vi "PH_AxisGUI_BaseClass.set Activity to GUI.vi"(4 "error in":errorcluster, 5 "no link":bool, 6 "Activity":T1, 7 "GUI Ref Activity":refnum<vi>) -> (0 "error out":errorcluster)   [LabVIEW 2014, in "PH_AxisGUI_BaseClass.lvlib"]
doc: "This VI sets the current activity to the GUI."
uses:
  PH_AxisGUI_BaseClass.lvlib
  PH_Stepmotor_BaseClass/PH_Stepmotor_BaseClass.Axis Activity.ctl
  PH_Stepmotor_BaseClass/PH_Stepmotor_BaseClass.lvlib
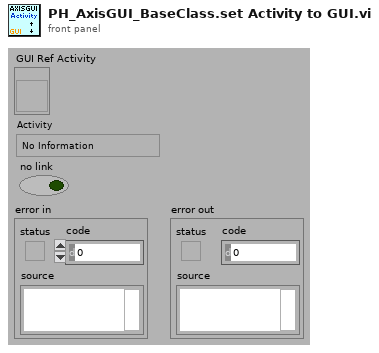
[diagram p1: front panel]
types:
  T1 = typedef "PH_Stepmotor_BaseClass.lvlib/PH_Stepmotor_BaseClass.Axis Activity.ctl" = enum16{"No Information", "stopped", "running", "Failure", "Alarm", "stopped at backward ES", "stopped at foreward ES"}
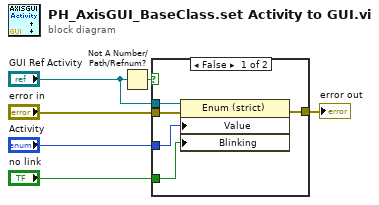
[diagram p0: block diagram]
diagram:
  n1 = Not A Number/Path/Refnum?(number/path/refnum="GUI Ref Activity") -> (NaN/Path/Refnum?=w6:bool)
  n2 = case shown="False" w6 {
    tunnel: "GUI Ref Activity" -> [w10 _]
    tunnel: [w11 w12] -> w2
    tunnel: "error in" -> [w9 w12]
    tunnel: "Activity" -> [w8 _]
    tunnel: "no link" -> [w7 _]
    frame False {
      n3 = property class="Enum (strict)"(reference=w10, error in=w9, "Value"=w8, "Blinking"=w7) -> (error out=w11:errorcluster)  [unwired: 1 out]
    }
    frame True {
    }
  }
  "error out" <- w2
